vi "Práctica3.vi"() -> ()   [LabVIEW 2024]
panel:
  out "String 2":string
  in  "String":string
  out "Boolean 2":bool
  in  "Boolean":bool
  out "Numeric 4":dbl
  out "Numeric 3":dbl
  in  "Numeric 2":dbl
  in  "Numeric":dbl
  # "Numéricos"
  # "Booleanos"
  # "De caracteres"
  # "Arreglos"
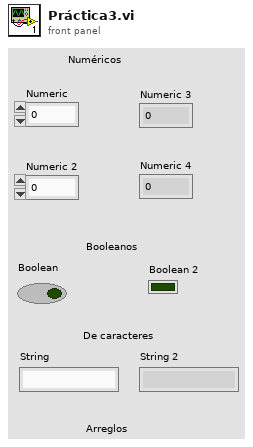
[diagram p1: front panel]
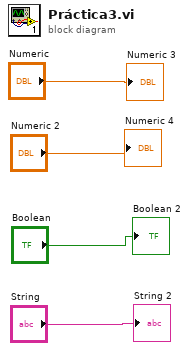
[diagram p0: block diagram]
diagram:
  "Numeric 3" <- "Numeric"
  "Numeric 4" <- "Numeric 2"
  "Boolean 2" <- "Boolean"
  "String 2" <- "String"
